vi "Tosca-Remap Signal Destinations.vi"(0 "Tosca":refnum<class "Parameters.lvclass">, 7 "FSM.Graph":refnum<class "FSM.Graph.lvclass">, 11 "error in (no error)":errorcluster) -> (4 "Tosca out":refnum<class "Parameters.lvclass">, 8 "FSM.Graph Out":refnum<class "FSM.Graph.lvclass">, 10 "remapped":bool, 15 "error IO":errorcluster)   [LabVIEW 2020]
uses:
  Classes/Parameters/Parameters.lvclass
  FSM Graph VIs/LV Source/Classes/FSM.Graph/FSM.Graph.lvclass
  Tosca-Globals.vi
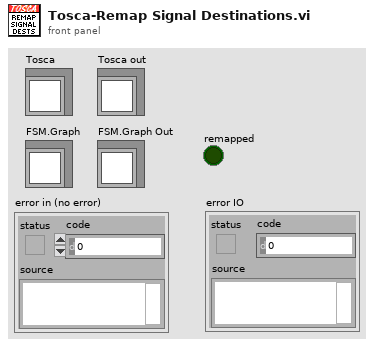
[diagram p1: front panel]
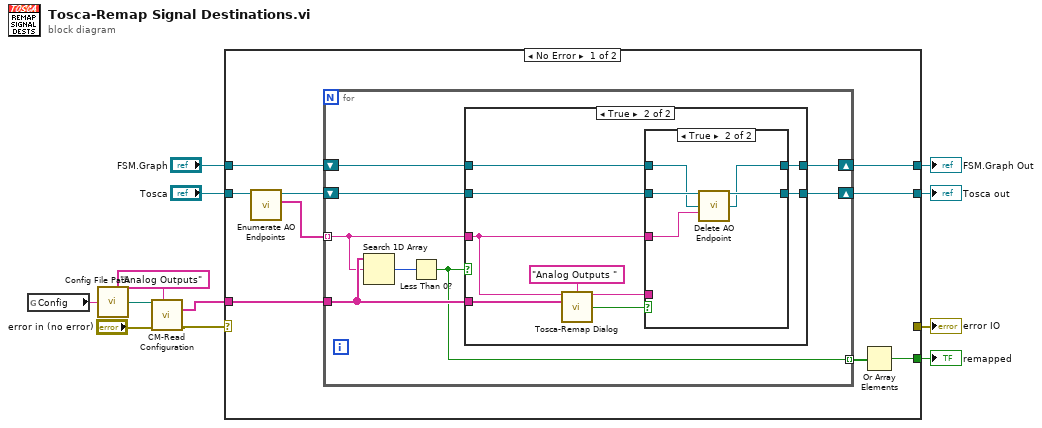
[diagram p0: block diagram]
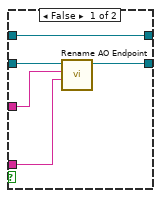
[diagram p3: hidden frame]
diagram:
  n1 = global read "Tosca-Globals.vi" "Config"() -> (w11:string)
  n2 = call "Config File Path.vi"("AppName"=w11) -> ("Default config file name"=w4:path)
  n3 = call "CM-Read Configuration.vi"("Connection File Path"=w4, "Section"="Analog Outputs", "error in (no error)"="error in (no error)") -> ("Names"=w1:string[], "error out"=w2:errorcluster)  [unwired: 8 in, 3 out]
  n4 = case shown="No Error" w2 {
    selector: w2 -> [_ w53]
    tunnel: w1 -> [w21 _]
    tunnel: [_ w53] -> w12
    tunnel: "Tosca" -> [w20 w52]
    tunnel: [w17 w52] -> w9
    tunnel: [w15 _] -> w8
    tunnel: "FSM.Graph" -> [w14 w51]
    tunnel: [w13 w51] -> w6
    frame No Error {
      n5 = call "Enumerate AO Endpoints.vi"("Tosca in"=w20) -> ("Endpoints"=w19:string[], "Tosca out"=w18:refnum<class "Parameters.lvclass">)  [unwired: 8 in, 1 out]
      n6 = for {
        tunnel: w21 -> [w29]
        tunnel: w19 -> [w27] mode=indexing
        shift-right: [w25] -> w17
        shift-left: w18 -> [w26]
        tunnel: [w24] -> w16 mode=indexing
        shift-right: [w22] -> w13
        shift-left: w14 -> [w23]
        n7 = Search 1D Array(1D array=w29, element=w27) -> (index of element=w28:i32)  [unwired: 1 in]
        n8 = Less Than 0?(x=w28) -> (x < 0?=w24:bool)
        n9 = case shown="True" w24 {
          tunnel: w29 -> [_ w39]
          tunnel: w27 -> [_ w35]
          tunnel: w26 -> [w31 w38]
          tunnel: [w31 w34] -> w25
          tunnel: w23 -> [w30 w33]
          tunnel: [w30 w32] -> w22
          frame False {
          }
          frame True {
            n10 = call "Tosca-Remap Dialog.vi"("Old Name In"=w35, "Type"="Analog Outputs ", "New Names"=w39) -> ("Old Name Out"=w36:string, "Deleted?"=w37:bool)  [unwired: 10 in, 1 out]
            n11 = case shown="True" w37 {
              tunnel: w38 -> [w45 w50]
              tunnel: w36 -> [w42 _]
              tunnel: w35 -> [w43 w49]
              tunnel: [w44 w48] -> w34
              tunnel: w33 -> [w41 w47]
              tunnel: [w41 w46] -> w32
              frame False {
                n12 = call "Rename AO Endpoint.vi"("New name"=w42, "Old name"=w43, "Tosca in"=w45) -> ("Tosca out"=w44:refnum<class "Parameters.lvclass">)  [unwired: 7 in, 1 out]
              }
              frame True {
                n13 = call "Delete AO Endpoint.vi"("Tosca in"=w50, "FSM.Graph"=w47, "Old name"=w49) -> ("Tosca out"=w48:refnum<class "Parameters.lvclass">, "FSM.Graph Out"=w46:refnum<class "FSM.Graph.lvclass">)  [unwired: 10 in, 1 out]
              }
            }
          }
        }
      }
      n14 = Or Array Elements(Boolean array=w16) -> (logical OR=w15:bool)
    }
    frame Error {
    }
  }
  "error IO" <- w12
  "Tosca out" <- w9
  "remapped" <- w8
  "FSM.Graph Out" <- w6
